vi "Service Request Enable Query.vi"(0 "VISA resource name":refnum<visa-resource-name>, 11 "error in (no error)":errorcluster) -> (4 "VISA resource name out":refnum<visa-resource-name>, 6 "Service Request Enable":T1, 15 "error out":errorcluster)   [LabVIEW 2020, in "eec EST 300.lvlib"]
doc: "Queries the Service Request enable register. Returns the decimal value of binary-weighted sum of bits.\n\nThe Standard Event Register consists of the following 8 bits.\nBit 0: MSB = Measurement Summary Bit\nBit 1: not used\nBit 2: EAV = Error Available \nBit 3: QSB = Questionable Summary Bit\nBit 4: MAV = Message Available\nBit 5: ESB = Event Summary Bit \nBit 6: not used\nBit 7: OSB = Operation Summary Bit\n\nExample:\n\nIf the query returns the binary mask (00000101|bin=5|dec) then SRQ(Service Request) is generated using is MAV and EAV only."
uses:
  <instrlib>/eec EST 300/eec EST 300.lvlib
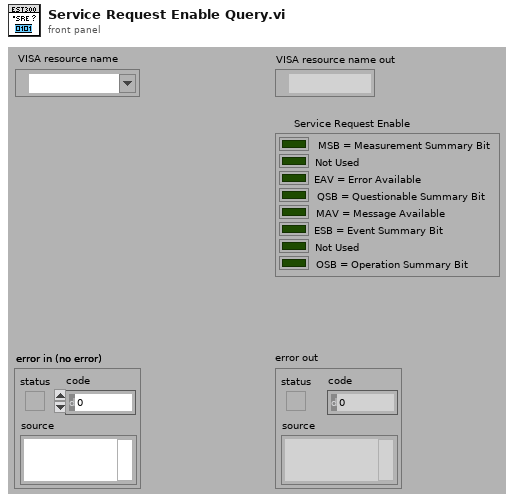
[diagram p1: front panel]
types:
  T1 = cluster{"MSB = Measurement Summary Bit":bool, "Not Used":bool, "EAV = Error Available":bool, "QSB = Questionable Summary Bit":bool, "MAV = Message Available":bool, "ESB = Event Summary Bit":bool, "Not Used":bool, "OSB = Operation Summary Bit":bool}
  T2 = cluster{"Boolean array[0]":bool, "Boolean array[1]":bool, "Boolean array[2]":bool, "Boolean array[3]":bool, "Boolean array[4]":bool, "Boolean array[5]":bool, "Boolean array[6]":bool, "Boolean array[7]":bool}
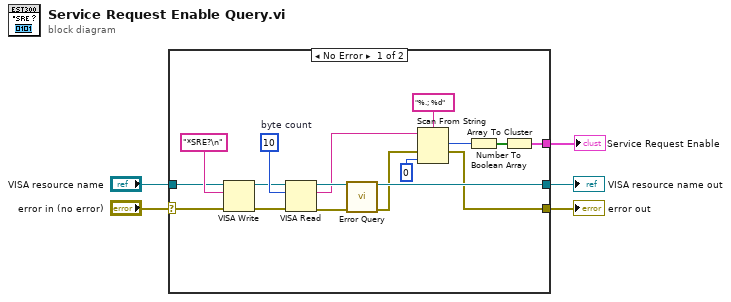
[diagram p0: block diagram]
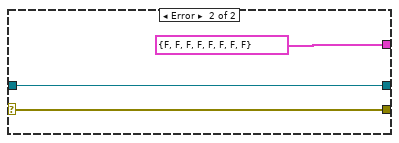
[diagram p2: hidden frame]
diagram:
  n1 = case shown="No Error" "error in (no error)" {
    selector: "error in (no error)" -> [w16 w25]
    tunnel: [w10 T2 {"Boolean array[0]"=FALSE, "Boolean array[1]"=FALSE, "Boolean array[2]"=FALSE, "Boolean array[3]"=FALSE, "Boolean array[4]"=FALSE, "Boolean array[5]"=FALSE, "Boolean array[6]"=FALSE, "Boolean array[7]"=FALSE} ("Boolean array")] -> w1
    tunnel: "VISA resource name" -> [w17 w24]
    tunnel: [w14 w24] -> w4
    tunnel: [w7 w25] -> w3
    frame No Error {
      w21 = u32 10  # byte count
      n2 = VISA Write(VISA resource name=w17, write buffer="*SRE?\n" ("Command to Send (empty)"), error in (no error)=w16) -> (VISA resource name out=w20:refnum<visa-resource-name>, error out=w19:errorcluster)  [unwired: 1 out]
      n3 = VISA Read(VISA resource name=w20, byte count=w21, error in (no error)=w19) -> (VISA resource name out=w13:refnum<visa-resource-name>, read buffer=w6:string, error out=w9:errorcluster)  [unwired: 1 out]
      n4 = call <instrlib>:"Error Query.vi"("VISA resource name"=w13, "error in (no error)"=w9) -> ("VISA resource name out"=w14:refnum<visa-resource-name>, "error out"=w8:errorcluster)  [unwired: 10 in, 2 out]
      n5 = Scan From String(format string="%.; %d" ("Format String"), input string=w6, error in=w8, default 1=u8 0 ("default value 1")) -> (offset past scan=w11:u32, error out=w7:errorcluster)  [unwired: 2 in, 1 out]
      n6 = Number To Boolean Array(number=w11) -> (Boolean array=w12:bool[])
      n7 = Array To Cluster(array=w12) -> (cluster=w10:T2)
    }
    frame Error {
    }
  }
  "error out" <- w3
  "VISA resource name out" <- w4
  "Service Request Enable" <- w1
